vi "RFInfo.vi"(0 "refnum":refnum<file>, 11 "offset":i32) -> (2 "RF Info":T1, 4 "dup refnum":refnum<file>, 6 "RF file name":string, 8 "RF file att":string, 10 "RF cal file name":string, 15 "RF cal file att":string)   [LabVIEW 2022 SP3]
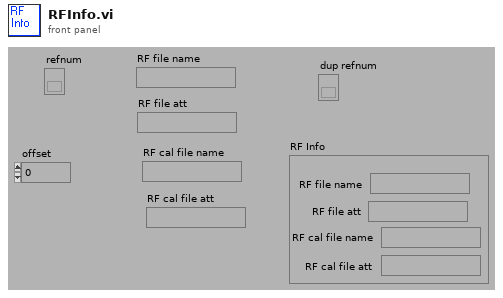
[diagram p1: front panel]
types:
  T1 = cluster{"RF file name":string, "RF file att":string, "RF cal file name":string, "RF cal file att":string}
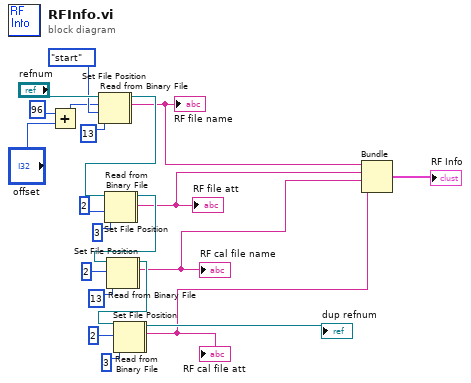
[diagram p0: block diagram]
diagram:
  n1 = Add(x=96 ("pos offset (0)"), y="offset") -> (x+y=w11:i32)
  n2 = Set File Position(offset (in bytes) (0)=w11, refnum="refnum", from (0:start)=enum16{"start", "end", "current"}."start" ("pos mode (0:2)")) -> (refnum out=w2:refnum<file>, error out=w1:errorcluster)  [unwired: 1 in]
  n3 = Read from Binary File(8:w1, 10:13 ("count"), 11:w2) -> (2:w16:string, 3:w24:refnum<file>)  [unwired: 5 out]
  "RF file name" <- w16
  n4 = Set File Position(refnum=w24, from (0:start)=2) -> (refnum out=w4:refnum<file>, error out=w3:errorcluster)  [unwired: 1 in, 1 out]
  n5 = Read from Binary File(8:w3, 10:3 ("count"), 11:w4) -> (2:w15:string, 3:w21:refnum<file>)  [unwired: 5 out]
  "RF file att" <- w15
  n6 = Set File Position(refnum=w21, from (0:start)=2) -> (refnum out=w6:refnum<file>, error out=w5:errorcluster)  [unwired: 1 in, 1 out]
  n7 = Read from Binary File(8:w5, 10:13 ("count"), 11:w6) -> (2:w14:string, 3:w17:refnum<file>)  [unwired: 5 out]
  "RF cal file name" <- w14
  n8 = Set File Position(refnum=w17, from (0:start)=2) -> (refnum out=w8:refnum<file>, error out=w7:errorcluster)  [unwired: 1 in, 1 out]
  n9 = Read from Binary File(8:w7, 10:3 ("count"), 11:w8) -> (2:w13:string, 3:→"dup refnum":refnum<file>)  [unwired: 5 out]
  "RF cal file att" <- w13
  n10 = Bundle(w16, w15, w14, w13) -> (→"RF Info":cluster{string, string, string, string})  [unwired: 1 out]
